vi "Array Functions.vi"() -> ()   [LabVIEW 2014]
panel:
  out "Subarray":i32[](array[numeric])
  out "2D Array (Integer)":i32[][](array[numeric])
  out "1D Array (DBL)":dbl[](array[numeric])
  out "2D Array Size":i32[](array[numeric])
  out "1D Array Size":i32
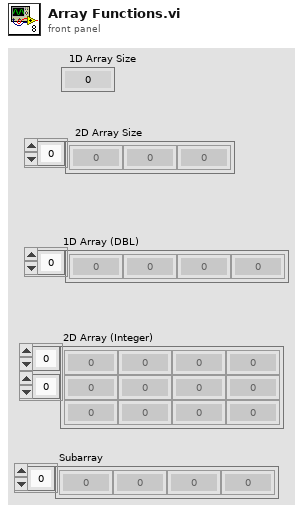
[diagram p1: front panel]
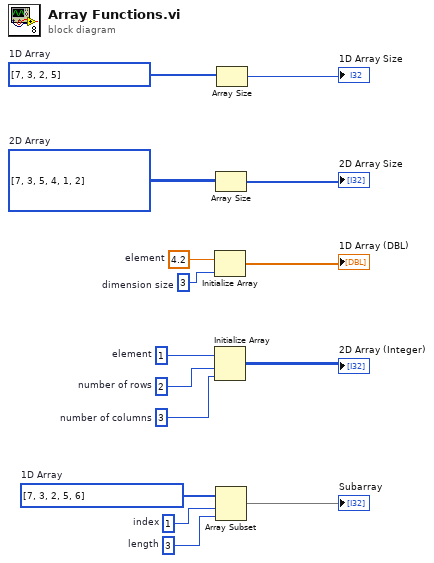
[diagram p0: block diagram]
diagram:
  w2 = 3  # length
  w3 = 1  # index
  w4 = i32[] [7, 3, 2, 5, 6]  # 1D Array
  w6 = 3  # number of columns
  w7 = 2  # number of rows
  w8 = 1  # element
  w10 = 3  # dimension size
  w11 = 4.2  # element
  w13 = i32[][] [[7, 3, 5], [4, 1, 2]]  # 2D Array
  w15 = i32[] [7, 3, 2, 5]  # 1D Array
  n1 = Initialize Array "Initialize Array"(w11, w10) -> (→"1D Array (DBL)":dbl[])
  n2 = Initialize Array "Initialize Array"(w8, w7, w6) -> (→"2D Array (Integer)":i32[][])
  n3 = Array Size(array=w13) -> (size(s)=→"2D Array Size":i32[])
  n4 = Array Subset "Array Subset"(array=w4, index=w3, length=w2) -> (→"Subarray":i32[])
  n5 = Array Size(array=w15) -> (size(s)=→"1D Array Size":i32)
